vi "Retrieve_memory_3_folders.vi"   [LabVIEW 2015]
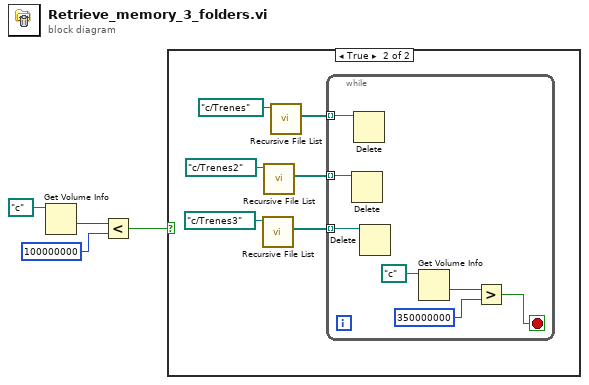
[diagram p0: block diagram]
diagram:
  n1 = Get Volume Info(11:path "c:/" ("path")) -> (1:w3:i64)  [unwired: 1 in, 5 out]
  n2 = Less?(x=w3, y=i64 100000000) -> (x < y?=w1:bool)
  n3 = case shown="True" w1 {
    frame False {
    }
    frame True {
      n4 = call <vilib>:"Recursive File List.vi"("Folder Path"=path "c:/Trenes3") -> ("All Files in Dir"=w9:path[])  [unwired: 6 in, 4 out]
      n5 = call <vilib>:"Recursive File List.vi"("Folder Path"=path "c:/Trenes2") -> ("All Files in Dir"=w7:path[])  [unwired: 6 in, 4 out]
      n6 = call <vilib>:"Recursive File List.vi"("Folder Path"=path "c:/Trenes") -> ("All Files in Dir"=w5:path[])  [unwired: 6 in, 4 out]
      n7 = while {
        tunnel: w9 -> [w17] mode=indexing
        tunnel: w7 -> [w12] mode=indexing
        tunnel: w5 -> [w11] mode=indexing
        stop <- w13 stop-if-true
        n8 = Delete(path (use dialog)=w12) -> ()  [unwired: 4 in, 3 out]
        n9 = Delete(path (use dialog)=w11) -> ()  [unwired: 4 in, 3 out]
        n10 = Delete(path (use dialog)=w17) -> ()  [unwired: 4 in, 3 out]
        n11 = Get Volume Info(11:path "c:/" ("path")) -> (1:w15:i64)  [unwired: 1 in, 5 out]
        n12 = Greater?(x=w15, y=i64 350000000) -> (0:w13:bool)
      }
    }
  }
